vi "Create_Litho_Queue.vi"(8 "error in":errorcluster, 9 "lithography_Offsets":cluster{"X":dbl, "Y":dbl}, 10 "Pattern Data":T1, 11 "Application":refnum<k7>) -> (0 "error out":errorcluster)   [LabVIEW 2016]
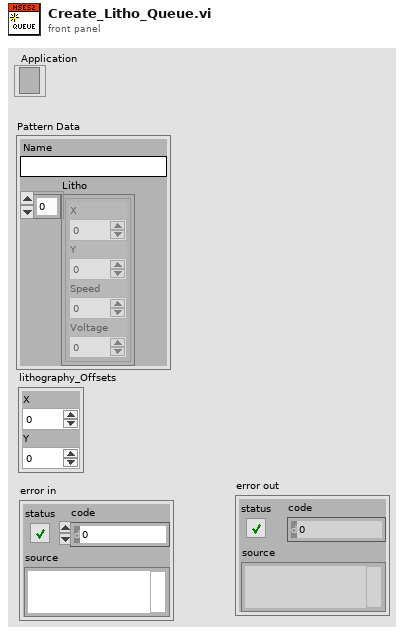
[diagram p1: front panel]
types:
  T1 = cluster{"Name":string, "Litho":cluster{"X":dbl, "Y":dbl, "Speed":dbl, "Voltage":dbl}[]}
  T2 = cluster{"X":dbl, "Y":dbl, "Speed":dbl, "Voltage":dbl}[]
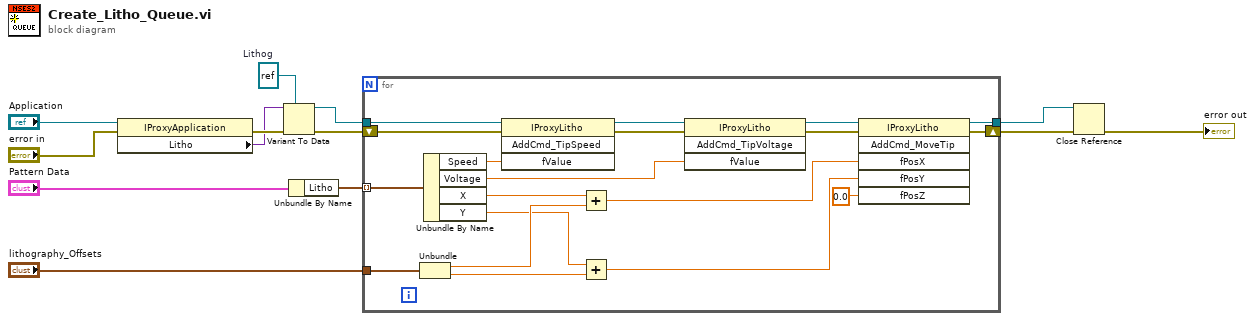
[diagram p0: block diagram]
diagram:
  w8 = refnum<k7> refnum  # Lithog
  n1 = property class="IProxyApplication"(reference="Application", error in="error in") -> (error out=w10:errorcluster, "Litho"=w9:variant)  [unwired: 1 out]
  n2 = Variant To Data(error in=w10, type=w8, Variant=w9) -> (data=w5:refnum<k7>, error out=w6:errorcluster)
  n3 = Unbundle By Name("Pattern Data") -> ("Litho"=w12:T2)
  n4 = for {
    shift-right: [w32] -> w3
    shift-left: w6 -> [w19]
    tunnel: w12 -> [w29] mode=indexing
    tunnel: "lithography_Offsets" -> [w28]
    tunnel: w5 -> [w16]
    tunnel: [w14] -> w1
    n5 = Unbundle(w28) -> ("X"=w27:dbl, "Y"=w24:dbl)
    n6 = Unbundle By Name(w29) -> ("Speed"=w17:dbl, "Voltage"=w23:dbl, "X"=w26:dbl, "Y"=w25:dbl)
    n7 = invoke class="IProxyLitho" method="AddCmd_TipSpeed"(reference=w16, error in=w19, "fValue"=w17) -> (reference out=w15:refnum<k7>, error out=w18:errorcluster)  [unwired: 1 in, 2 out]
    n8 = Add(x=w26, y=w27) -> (x+y=w31:dbl)
    n9 = Add(x=w25, y=w24) -> (x+y=w30:dbl)
    n10 = invoke class="IProxyLitho" method="AddCmd_TipVoltage"(reference=w15, error in=w18, "fValue"=w23) -> (reference out=w20:refnum<k7>, error out=w21:errorcluster)  [unwired: 1 in, 2 out]
    n11 = invoke class="IProxyLitho" method="AddCmd_MoveTip"(reference=w20, error in=w21, "fPosX"=w31, "fPosY"=w30, "fPosZ"=0.0 ("fPosX")) -> (reference out=w14:refnum<k7>, error out=w32:errorcluster)  [unwired: 1 in, 4 out]
  }
  n12 = Close Reference(reference=w1, error in (no error)=w3) -> (error out=→"error out":errorcluster)
